vi "Event Messenger Channel Lesson 4b (wrong way).vi"() -> ()   [LabVIEW 2019]
doc: "Lesson 4b shows the wrong way to have one Event Messenger channel wire trigger two separate Event structures. <b>This VI will abort when run.</b>"
uses:
  <extravilib>/ChannelInstances/Event Messenger-i32/Instantiate.vi
  <extravilib>/ChannelInstances/Event Messenger-i32/))Channel.vi
  <extravilib>/ChannelInstances/Event Messenger-i32.lvlib
panel:
  out "Consumer Beta":i32
  out "Producer":i32
  out "Consumer Alpha":i32
  in  "Stop":bool
  # "Overview: This VI demonstrates how to use the Event Messenger channel wire.\n\nLesson 4b shows the wrong way to have one Event Messenger channel wire trigger two separate Event structures. This VI will abort when run.\n\nInstructions:\n1. Run the VI. \nThe VI will immediately stop itself and report an error. This is an example of what NOT to do. Refer to lesson 4a for the right way to do this.\n2. Open the block diagram. Review the comments there to see how this VI works."
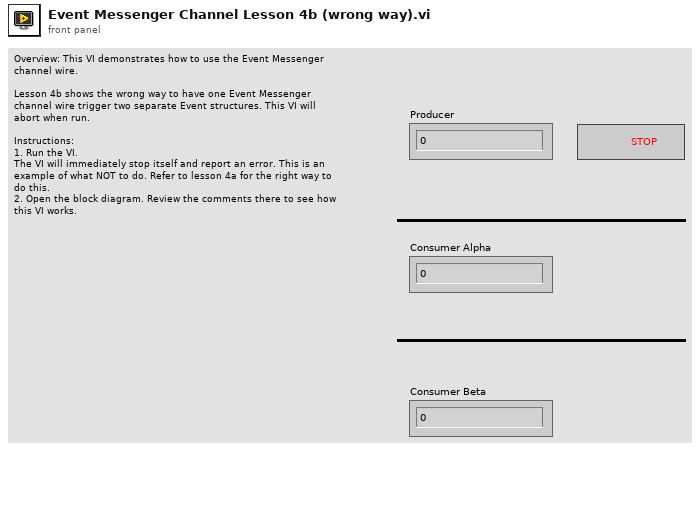
[diagram p1: front panel]
types:
  T1 = typedef "Event Messenger-i32.lvlib/))Channel.ctl" = refnum<queue>
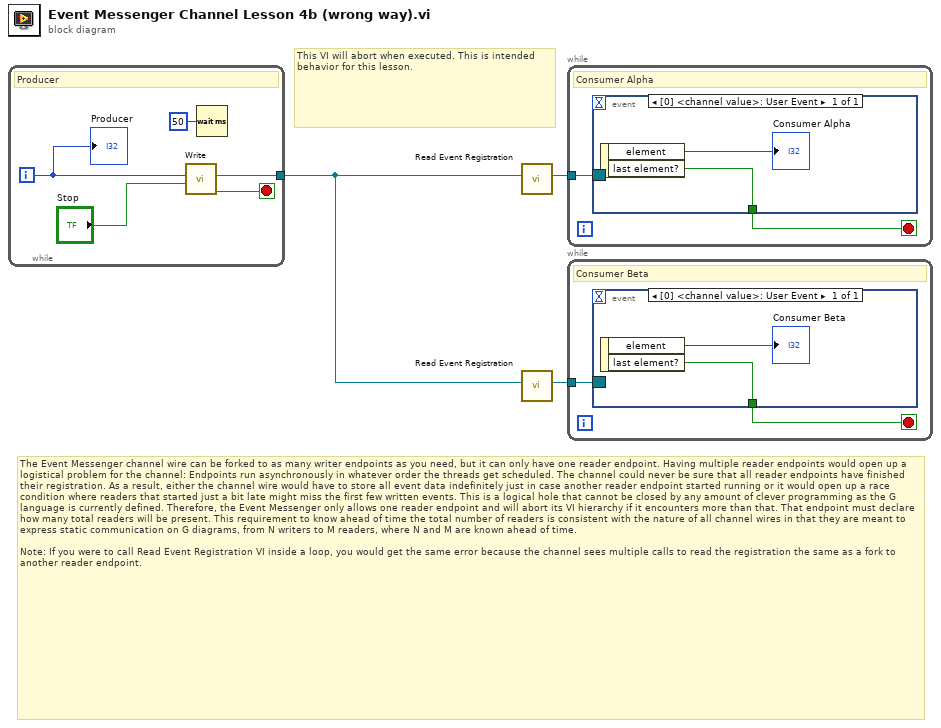
[diagram p0: block diagram]
diagram:
  # "This VI will abort when executed. This is intended behavior for this lesson."
  # "The Event Messenger channel wire can be forked to as many writer endpoints as you need, but it can only have one reader endpoint. Having multiple reader endpoints would open up a logistical problem for the channel: Endpoints run asynchronously in whatever order the threads get scheduled. The channel could never be sure that all reader endpoints have finished their registration. As a result, either the channel wire would have to store all event data indefinitely just in case another reader endpoint started running or it would open up a race condition where readers that started just a bit late might miss the first few written events. This is a logical hole that cannot be closed by any amount of clever programming as the G language is currently defined. Therefore, the Event Messenger only allows one reader endpoint and will abort its VI hierarchy if it encounters more than that. That endpoint must declare how many total readers will be present. This requirement to know ahead of time the total number of readers is consistent with the nature of all channel wires in that they are meant to express static communication on G diagrams, from N writers to M readers, where N and M are known ahead of time. \n\nNote: If you were to call Read Event Registration VI inside a loop, you would get the same error because the channel sees multiple calls to read the registration the same as a fork to another reader endpoint."
  n1 = while {
    tunnel: [w5] -> w3
    i -> [w8]
    stop <- w7 stop-if-true
    # "Producer"
    n2 = call <extravilib>:"Write.vi"("last element? (F)"="Stop", "element"=w8) -> ("done?"=w7:bool, "channel"=w5:T1)  [unwired: 8 in]
    n3 = Wait (ms)(milliseconds to wait=u32 50) -> ()  [unwired: 1 out]
    "Producer" <- w8
  }
  n4 = call <extravilib>:"Read Event Registration.vi"("channel"=w3) -> ("event registration refnum"=w2:refnum<event-registration>)  [unwired: 10 in]
  n5 = call <extravilib>:"Read Event Registration.vi"("channel"=w3) -> ("event registration refnum"=w1:refnum<event-registration>)  [unwired: 10 in]
  n6 = while {
    tunnel: w2 -> [w10]
    stop <- w9 stop-if-true
    # "Consumer Alpha"
    n7 = event shown="[0] <channel value>: User Event" {
      selector: w10 -> [_]
      dyn-events: _ -> [_]
      timeout: _ -> [_]
      tunnel: [w11] -> w9
      event User Event {
        n8 = event-data() -> ("element"=→"Consumer Alpha":i32, "last element?"=w11:bool)  [unwired: 1 in]
      }
    }
  }
  n9 = while {
    tunnel: w1 -> [w14]
    stop <- w13 stop-if-true
    # "Consumer Beta"
    n10 = event shown="[0] <channel value>: User Event" {
      selector: w14 -> [_]
      dyn-events: _ -> [_]
      timeout: _ -> [_]
      tunnel: [w16] -> w13
      event User Event {
        n11 = event-data() -> ("element"=→"Consumer Beta":i32, "last element?"=w16:bool)  [unwired: 1 in]
      }
    }
  }
